vi "Configuration - Determine Device Type.vi"(10 "Type String In":string) -> (2 "Device Type Out":T1)   [LabVIEW 2017, in "Communications Library.lvlib"]
uses:
  Communications Library.lvlib
  Typedefs/DTACQ Device Type--Enum.ctl
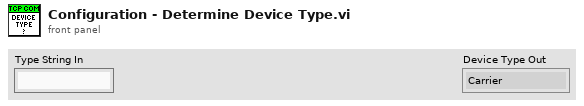
[diagram p1: front panel]
types:
  T1 = typedef "Communications Library.lvlib/DTACQ Device Type--Enum.ctl" = enum16{"Carrier", "Analog In Module", "Analog Out Module", "Generic Module"}
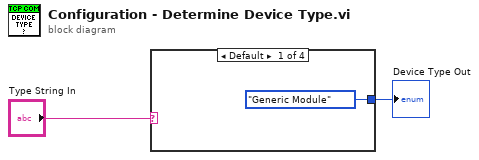
[diagram p0: block diagram]
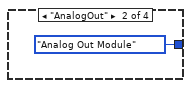
[diagram p2: hidden frame]
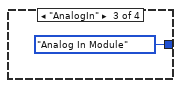
[diagram p3: hidden frame]
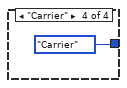
[diagram p4: hidden frame]
diagram:
  n1 = case shown="Default" "Type String In" {
    tunnel: [DTACQ_Device_Type--Enum."Generic Module" ("Device Type") DTACQ_Device_Type--Enum."Analog Out Module" ("Device Type") DTACQ_Device_Type--Enum."Analog In Module" ("Device Type") DTACQ_Device_Type--Enum."Carrier" ("Device Type")] -> w2
    frame Default {
    }
    frame "AnalogOut" {
    }
    frame "AnalogIn" {
    }
    frame "Carrier" {
    }
  }
  "Device Type Out" <- w2
